vi "State_Machine.vi"(8 "error in (no error)":errorcluster caption="entrée d'erreur (pas d'erreur)", 11 "Delay en entrée":refnum<class "P2201_Scan_Screen.lvclass">) -> (0 "error out":errorcluster caption="sortie d'erreur", 2 "Json_String":string, 3 "Delay en sortie":refnum<class "P2201_Scan_Screen.lvclass">)   [LabVIEW 2020, in "Library Test.lvlib" / "P2201_Scan_Screen.lvclass"]
uses:
  P2201_Scan_Screen.lvclass
  C:/Users/ngarcin/OneDrive - Altyor/Standard TB/Suite TB45/Class/Test/Test (Default)/Test (Default).lvclass
  Popup/Class Popup Operator_Input Batch_AIS/Class Popup Operator_Input_PCRE.lvclass
  Popup/Class Popup (Main)/Class Popup (Main).lvclass
  Commun VI/TypeDef/Variable Printable.ctl
  JSON API/JSON Value/Set from JSON string.vi
  JSON API/JSON Value/JSON Value.lvclass
  JSON API/Variant JSON/Variant JSON.lvlib
  JSON API/Get Polymorphic/JSON GetSet.lvlib
  Commun VI/Library Commun.lvlib
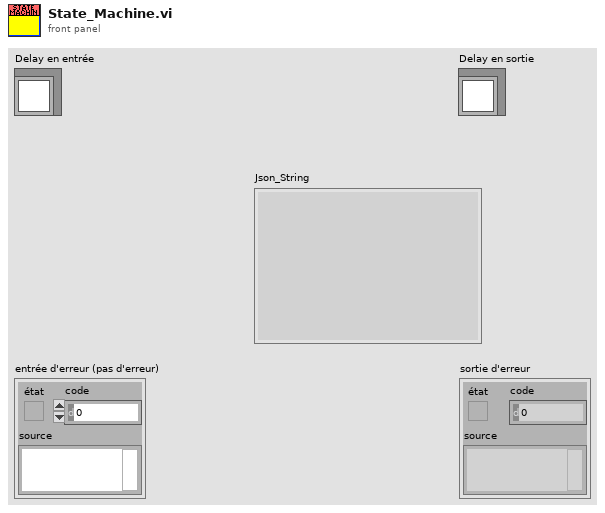
[diagram p1: front panel]
types:
  T1 = typedef "Variable Printable.ctl" = string
  T2 = enum16{"Get Variable", "Get All Variables", "Set Variable", "Delete Variable", "Delete All Variable"}
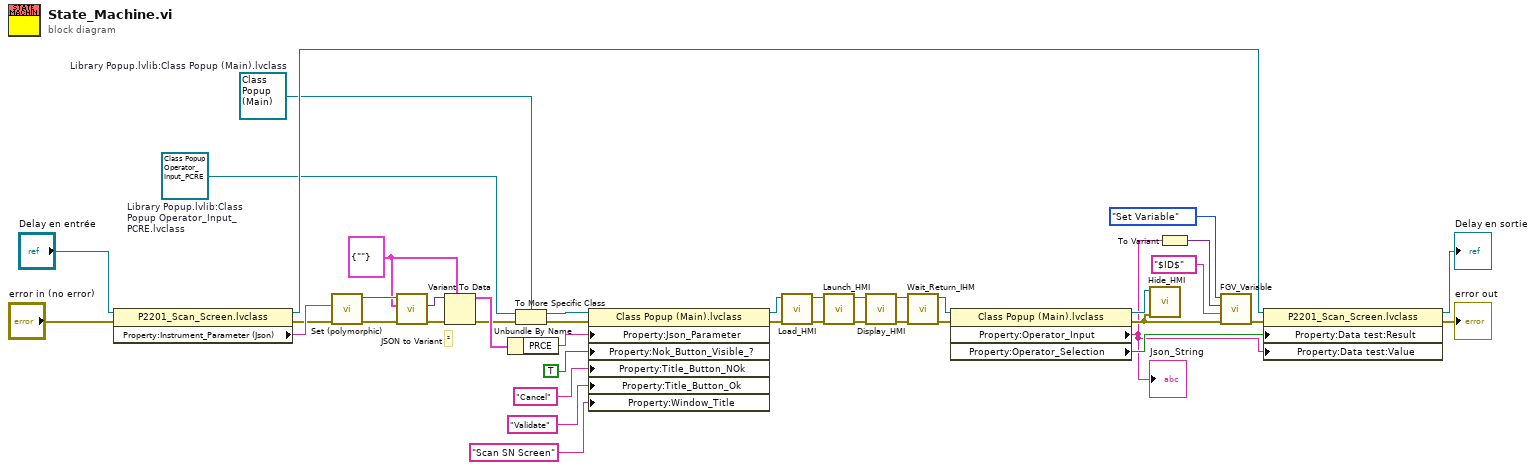
[diagram p0: block diagram]
diagram:
  w13 = refnum<class "Class Popup (Main).lvclass"> refnum  # Library Popup.lvlib:Class Popup (Main).lvclass
  w16 = cluster{"PRCE":string} {"PRCE"=""}
  w12 = refnum<class "Class Popup Operator_Input_PCRE.lvclass"> refnum  # Library Popup.lvlib:Class Popup Operator_Input_PCRE.lvclass
  # "²"
  n1 = property class="P2201_Scan_Screen.lvclass"(reference="Delay en entrée", error in="error in (no error)") -> (reference out=w22:refnum<class "P2201_Scan_Screen.lvclass">, error out=w38:errorcluster, "Property:Instrument_Parameter (Json)"=w40:string)
  n2 = call-poly "Set (polymorphic).vi"("error in (no error)"=w38, "JSON stream"=w40) -> ("error out"=w18:errorcluster, "JSON Value out"=w20:refnum<class "JSON Value.lvclass">)  [unwired: 7 in, 1 out]
  n3 = call "JSON to Variant.vi"("error in (no error)"=w18, "Variant (Data Type)"=w16, "JSON Value"=w20) -> ("error out"=w19:errorcluster, "Variant out"=w17:variant)  [unwired: 7 in]
  n4 = Variant To Data(error in=w19, type=w16, Variant=w17) -> (data=w15:cluster{"PRCE":string}, error out=w10:errorcluster)
  n5 = Unbundle By Name(w15) -> ("PRCE"=w14:string)
  n6 = To More Specific Class(target class=w13, reference=w12, error in=w10) -> (specific class reference=w11:refnum<class "Class Popup (Main).lvclass">, error out=w9:errorcluster)
  n7 = property class="Class Popup (Main).lvclass"(reference=w11, error in=w9, "Property:Json_Parameter"=w14, "Property:Nok_Button_Visible_?"=TRUE ("Nok_Button_Visible_?"), "Property:Title_Button_NOk"="Cancel" ("Title_Button_NOk"), "Property:Title_Button_Ok"="Validate" ("Title_Button_Ok"), "Property:Window_Title"="Scan SN Screen" ("Window_Title")) -> (reference out=w32:refnum<class "Class Popup (Main).lvclass">, error out=w31:errorcluster)
  n8 = call-dynamic "Load_HMI.vi"("error in (no error)"=w31, "Class Popup (Default) en entrée"=w32) -> ("error out"=w37:errorcluster, "Class Popup (Default) en sortie"=w36:refnum<class "Class Popup (Main).lvclass">)  [unwired: 8 in]
  n9 = call-dynamic "Launch_HMI.vi"("error in (no error)"=w37, "Class Popup (Default) en entrée"=w36) -> ("error out"=w35:errorcluster, "Class Popup (Default) en sortie"=w34:refnum<class "Class Popup (Main).lvclass">)  [unwired: 8 in]
  n10 = call-dynamic "Display_HMI.vi"("error in (no error)"=w35, "Class Popup (Default) en entrée"=w34) -> ("error out"=w7:errorcluster, "Class Popup (Default) en sortie"=w33:refnum<class "Class Popup (Main).lvclass">)  [unwired: 8 in]
  n11 = call-dynamic "Wait_Return_IHM.vi"("error in (no error)"=w7, "Class Popup (Default) en entrée"=w33) -> ("error out"=w8:errorcluster, "Class Popup (Default) en sortie"=w27:refnum<class "Class Popup (Main).lvclass">)  [unwired: 8 in]
  n12 = property class="Class Popup (Main).lvclass"(reference=w27, error in=w8) -> (reference out=w26:refnum<class "Class Popup (Main).lvclass">, error out=w3:errorcluster, "Property:Operator_Input"=w1:string, "Property:Operator_Selection"=w21:bool)
  "Json_String" <- w1
  n13 = call-dynamic "Hide_HMI.vi"("error in (no error)"=w3, "Class Popup (Default) en entrée"=w26) -> ()  [unwired: 8 in, 2 out]
  n14 = To Variant(anything=w1) -> (Variant=w6:variant)
  n15 = call "FGV_Variable.vi"("error in (no error)"=w3, "Variable"=T1 "$ID$", "Data In"=w6, "Function"=T2."Set Variable") -> ("error out"=w2:errorcluster)  [unwired: 5 in, 2 out]
  n16 = property class="P2201_Scan_Screen.lvclass"(reference=w22, error in=w2, "Property:Data test:Result"=w21, "Property:Data test:Value"=w1) -> (reference out=→"Delay en sortie":refnum<class "P2201_Scan_Screen.lvclass">, error out=→"error out":errorcluster)
